vi "sim spectrum.vi"(6 "y":dbl[](array[numeric])=array[4097 elements], 7 "npars":u32, 8 "error in (no error)":errorcluster, 9 "pars":dbl[](array[numeric])=array[4097 elements], 10 "npts":u32, 11 "B":dbl[](array[numeric])=array[4097 elements]) -> (0 "error out":errorcluster, 2 "npts out":u32, 4 "y out":dbl[](array[numeric]), 5 "npars out":u32)   [LabVIEW 2016, in "libFitSpectraLabview_Rev5.lvlib"]
doc: "void FIT_LABVIEW_API sim_spectrum(const double *B, unsigned int *npts,\n const double *pars, unsigned int *npars, double *y);"
uses:
  libFitSpectraLabview_Rev5.lvlib
  Documents/Software/Labview Fitting/LabviewCompiled/Rev5/libFitSpectraLabview_Rev5.dll
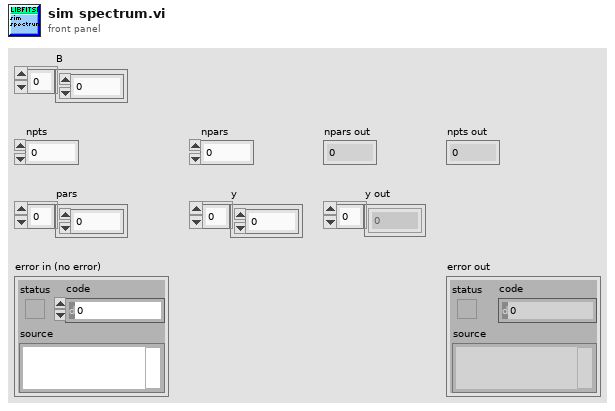
[diagram p1: front panel]
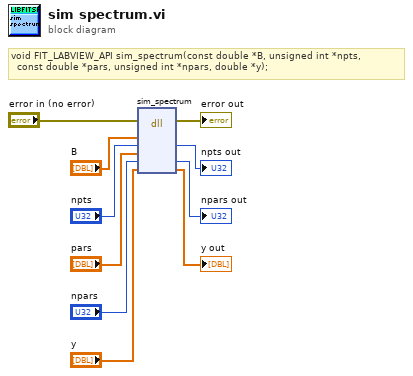
[diagram p0: block diagram]
diagram:
  # "void FIT_LABVIEW_API sim_spectrum(const double *B, unsigned int *npts,\n  const double *pars, unsigned int *npars, double *y);"
  n1 = dll-call lib="C:/Users/Wilson Schreiber/Documents/Software/Labview Fitting/LabviewCompiled/Rev5/libFitSpectraLabview_Rev5.*" fn="sim_spectrum"(error in="error in (no error)", "B"="B", "npts"="npts", "pars"="pars", "npars"="npars", "y"="y") -> (error out=→"error out":errorcluster, "npts"=→"npts out":u32, "npars"=→"npars out":u32, "y"=→"y out":dbl[])  [unwired: 5 in, 1 out]
